vi "Byte Buffer.Allocate.vi"(8 "error in (no error)":errorcluster, 11 "bytes to allocate":i32) -> (0 "error out":errorcluster, 3 "buffer":string)   [LabVIEW 2016, in "VeriStand Data.lvlib" / "Byte Buffer.lvclass"]
doc: "Allocates a new string buffer of size <B>bytes to allocate</B>."
uses:
  Byte Buffer.lvclass
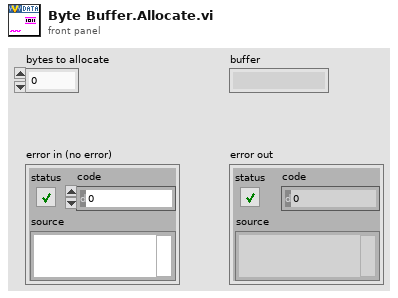
[diagram p1: front panel]
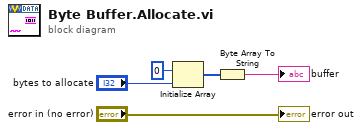
[diagram p0: block diagram]
diagram:
  n1 = Initialize Array(u8 0 ("element"), "bytes to allocate") -> (w3:u8[])
  n2 = Byte Array To String(unsigned byte array=w3) -> (string=→"buffer":string)
  "error out" <- "error in (no error)"
